vi "GT Go Home.vi"(8 "error in (no error)":errorcluster caption="错误输入（无错误）", 9 "pHomePrm":T1 {"mode" items=["LIMIT (10)：限位回原点"=10, "LIMIT_HOME (11)：限位+Home回原点"=11, "LIMIT_INDEX (12)：限位+Index回原点"=12, "LIMIT_HOME_INDEX (13)：限位+Home+Index回原点"=13, "HOME (20)：Home回原点"=20, "HOME_INDEX (22)：Home+Index回原点"=22, "INDEX (30)：Index回原点"=30, "FORCED_HOME (40)：强制Home回原点"=40, "FORCED_HOME_INDEX (41)：强制Home+Index回原点"=41]}, 10 "axis":i16, 11 "cardNum":i16) -> (0 "error out":errorcluster caption="错误输出", 3 "function return":i16)   [LabVIEW 2020, in "gts.lvlib"]
doc: "GT_API GT_GoHome(short cardNum,short axis,THomePrm *pHomePrm);"
uses:
  gts.lvlib
  Controls/HomePrm.ctl
  Controls/HomeMode.ctl
  dll/32bit/multi_card/gts.dll
  Controls/Controls.lvlib
panel:
  # "typedef struct  \n{\n\tshort mode;\t\t\t\t\t\t// 回零模式\n\tshort moveDir;\t\t\t\t\t// 设置启动搜索时的运动方向\n\tshort indexDir;\t\t\t\t\t// 设置Index搜索方向\n\tshort edge;\t\t\t\t\t\t// 设置捕获沿\n\tshort triggerIndex;\t\t\t\t// 用于设置触发器，为-1表示和轴号对应\n\tshort pad1[3];\t\t\t\t\t// 保留1\n\tdouble velHigh;\t\t\t\t\t// Home搜索速度\n\tdouble velLow;\t\t\t\t\t// Index搜索速度\n\tdouble acc;\t\t\t\t\t\n\tdouble dec;\n\tshort smoothTime;\n\tshort pad2[3];\t\t\t\t\t// 保留2\n\tlong homeOffset;\t\t\t\t// 原点偏移\n\tlong searchHomeDistance;\t\t// Home最大搜索距离，为0表示不限制\n\tlong searchIndexDistance;\t\t// Index最大搜索距离，为0表示不限制\n\tlong escapeStep;\t\t\t\t// 脱离步长\n\tlong pad3[2];\t\t\t\t\t// 保留3\n} THomePrm;"
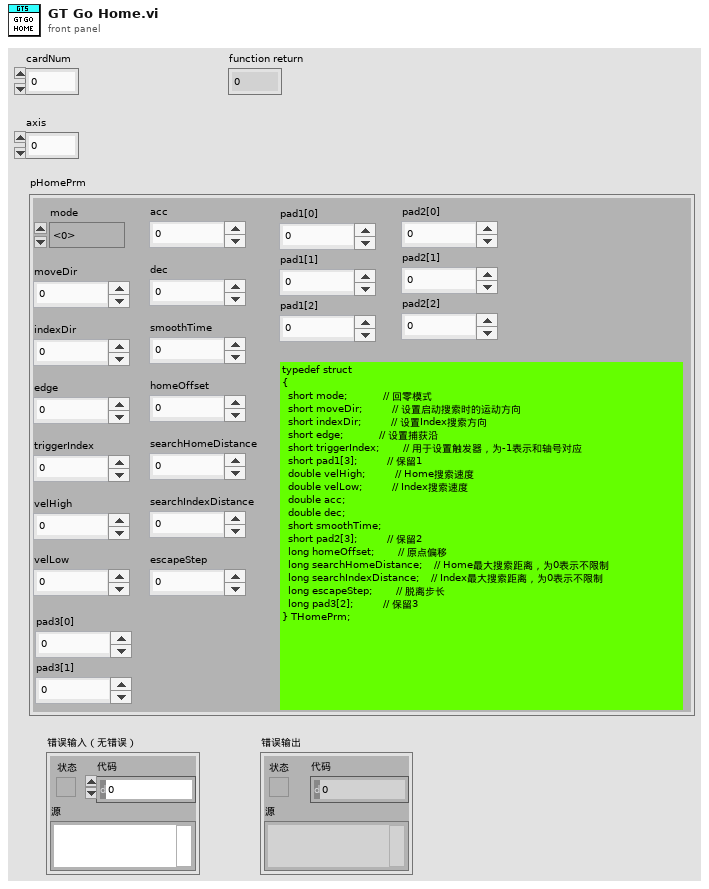
[diagram p1: front panel]
types:
  T1 = typedef "Controls.lvlib/HomePrm.ctl" = cluster{"mode":T2, "moveDir":i16, "indexDir":i16, "edge":i16, "triggerIndex":i16, "pad1[0]":i16, "pad1[1]":i16, "pad1[2]":i16, "velHigh":dbl, "velLow":dbl, "acc":dbl, "dec":dbl, "smoothTime":i16, "pad2[0]":i16, "pad2[1]":i16, "pad2[2]":i16, "homeOffset":i32, "searchHomeDistance":i32, "searchIndexDistance":i32, "escapeStep":i32, "pad3[0]":i32, "pad3[1]":i32}
  T2 = typedef "Controls.lvlib/HomeMode.ctl" = u8
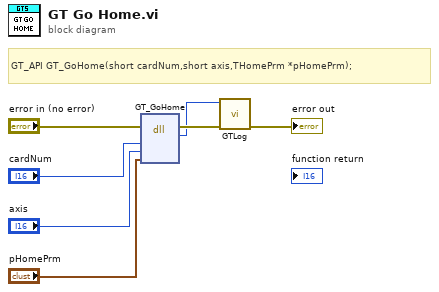
[diagram p0: block diagram]
diagram:
  # "GT_API GT_GoHome(short cardNum,short axis,THomePrm *pHomePrm);"
  n1 = dll-call lib="C:/1228/dll/32bit/multi_card/gts.dll" fn="GT_GoHome"(error in="error in (no error)", "cardNum"="cardNum", "axis"="axis", "pHomePrm"="pHomePrm") -> (error out=w3:errorcluster, w1:i16)  [unwired: 5 in, 1 out]
  n2 = call "GTLog.vi"("error in (no error)"=w3, "Numeric"=w1) -> ("error out"=→"error out":errorcluster)  [unwired: 9 in]
